vi "TeamLookUP.vi"() -> ()   [LabVIEW 2016]
panel:
  in  "Previous":bool
  in  "Next":bool
  out "Image":T1(plugin-control)
  out "Data":string
  out "Location":string
  out "Name":string
  in  "Done":bool
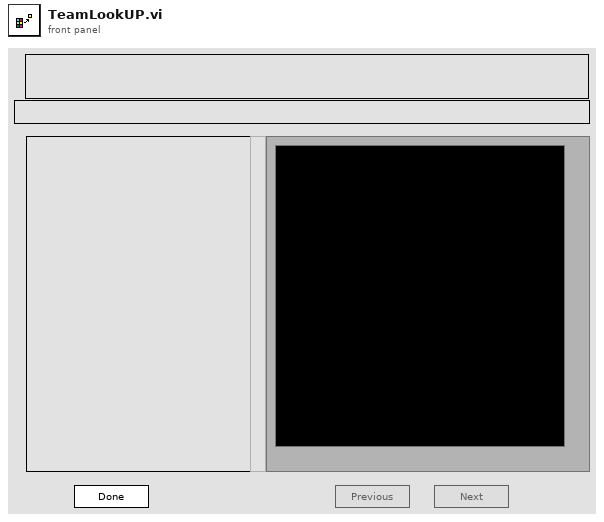
[diagram p1: front panel]
types:
  T1 = typedef "IMAQ Image.ctl" = refnum<image>
  T2 = typedef "Image Type" = u32
  T3 = enum8{"Enabled", "Disabled", "Disabled and Grayed Out"}
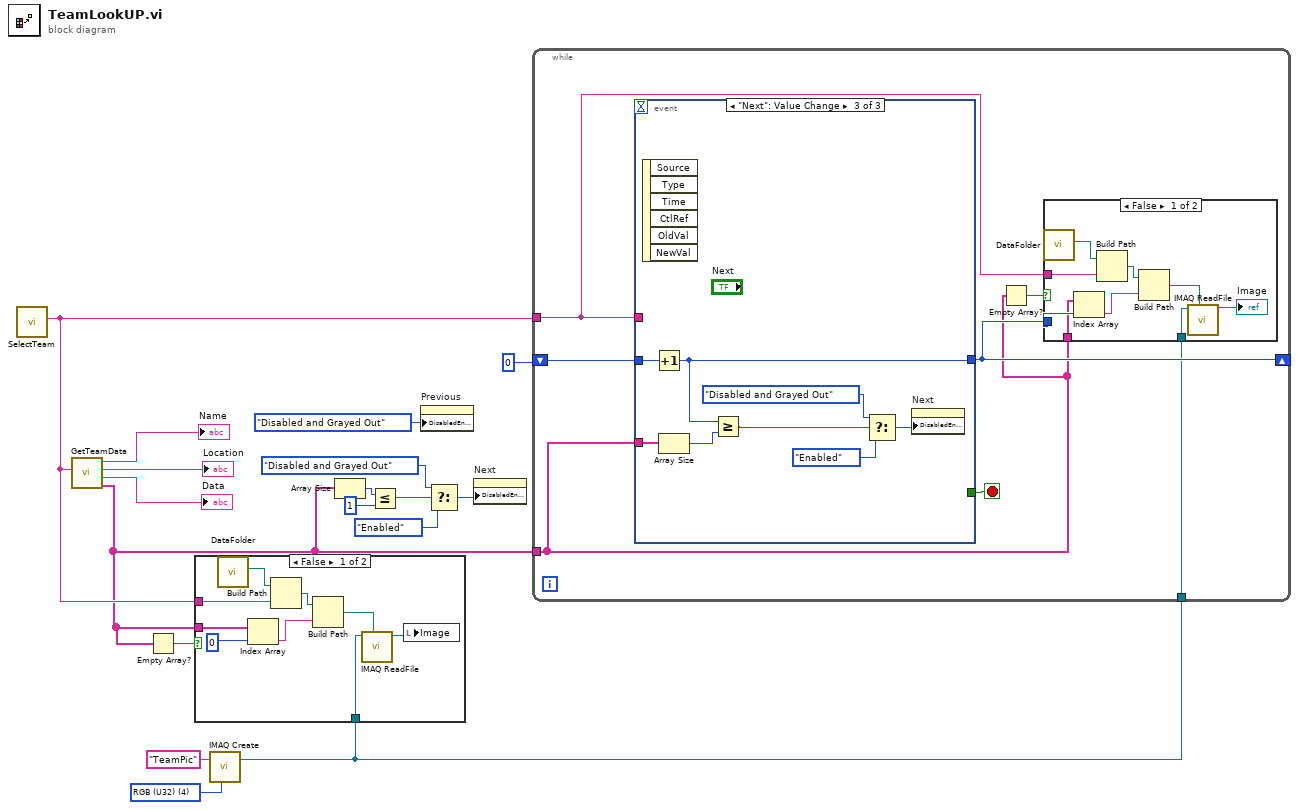
[diagram p0: block diagram]
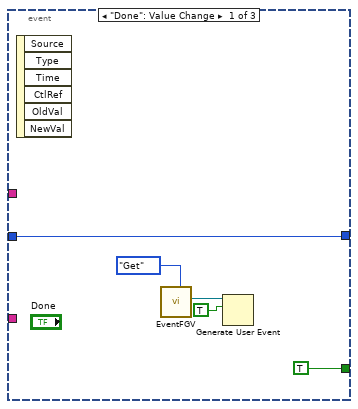
[diagram p4: hidden frame]
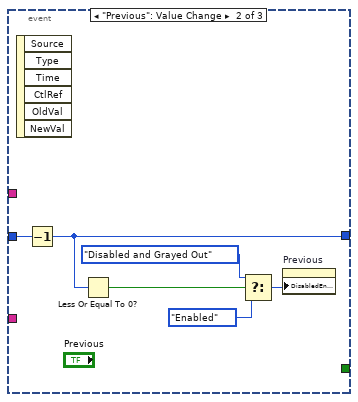
[diagram p5: hidden frame]
diagram:
  w5 = T2 4 items=["Grayscale (U8)", "Grayscale (I16)", "Grayscale (SGL)", "Complex (CSG)", "RGB (U32)", "HSL (U32)", "RGB (U64)", "Grayscale (U16)"] ("Image Type")
  n1 = call "SelectTeam.vi"() -> ("Selected Team"=w4:string)  [unwired: 11 in]
  n2 = call "GetTeamData.vi"("Team #"=w4) -> ("Pictures"=w2:string[], "Data"=→"Data":string, "Location"=→"Location":string, "Name"=→"Name":string)  [unwired: 7 in]
  n3 = Empty Array?(array=w2) -> (empty?=w3:bool)
  n4 = call "IMAQ Create"("Image Name"="TeamPic", "Image Type"=w5) -> ("New Image"=w1:T1)  [unwired: 3 in, 1 out]
  n5 = case shown="False" w3 {
    tunnel: w2 -> [w22 _]
    tunnel: w4 -> [w20 _]
    tunnel: w1 -> [w18 _]
    frame False {
      n6 = call "DataFolder.vi"() -> ("appended path"=w23:path)  [unwired: 11 in]
      n7 = Index Array(array=w22, index=0) -> (element=w25:string)
      n8 = Build Path(base path=w23, name or relative path=w20) -> (appended path=w24:path)
      n9 = Build Path(base path=w24, name or relative path=w25) -> (appended path=w26:path)
      n10 = call "IMAQ ReadFile"("File Path"=w26, "Image"=w18) -> ("Image Out"=w19:T1)  [unwired: 5 in, 4 out]
      n11 = local write "Image"(w19) -> ()
    }
    frame True {
    }
  }
  n12 = Array Size(array=w2) -> (size(s)=w12:i32)
  n13 = Less Or Equal?(x=w12, y=1) -> (x <= y?=w9:bool)
  n14 = property on="Previous" class="Bool"("DisabledEnum"=T3."Disabled and Grayed Out" ("Disabled")) -> ()  [unwired: 2 in, 2 out]
  n15 = Select(t=T3."Disabled and Grayed Out" ("Disabled"), s=w9, f=T3."Enabled" ("Disabled")) -> (s? t:f=w10:T3)
  n16 = property on="Next" class="Bool"("DisabledEnum"=w10) -> ()  [unwired: 2 in, 2 out]
  n17 = while {
    tunnel: w4 -> [w30]
    shift-right: [w31] -> _
    shift-left: 0 -> [w32]
    tunnel: w2 -> [w28]
    tunnel: w1 -> [w29]
    stop <- w33 stop-if-true
    n18 = event shown="[2] \"Next\": Value Change" {
      selector: _ -> [_ _ _]
      dyn-events: _ -> [_ _ _]
      timeout: _ -> [_ _ _]
      tunnel: [TRUE _ _] -> w33
      tunnel: w30 -> [_ _ _]
      tunnel: [w43 w52 w57] -> w31
      tunnel: w32 -> [w43 w53 w61]
      tunnel: w28 -> [_ _ w56]
      event "Done": Value Change {
        n19 = event-data() -> ()  [unwired: 1 in, 6 out]
        n20 = call "EventFGV.vi"("Action"=enum16{"Set", "Get"}."Get") -> ("user event out"=w47:refnum<user-event>)  [unwired: 10 in]
        n21 = Generate User Event(user event=w47, event data cluster=TRUE ("event data")) -> ()  [unwired: 2 in, 2 out]
      }
      event "Previous": Value Change {
        n22 = event-data() -> ()  [unwired: 1 in, 6 out]
        n23 = Decrement(x=w53) -> (x-1=w52:i32)
        n24 = Less Or Equal To 0?(x=w52) -> (x <= 0?=w48:bool)
        n25 = Select(t=T3."Disabled and Grayed Out" ("Disabled"), s=w48, f=T3."Enabled" ("Disabled")) -> (s? t:f=w49:T3)
        n26 = property on="Previous" class="Bool"("DisabledEnum"=w49) -> ()  [unwired: 2 in, 2 out]
      }
      event "Next": Value Change {
        n27 = event-data() -> ()  [unwired: 1 in, 6 out]
        n28 = Increment(x=w61) -> (x+1=w57:i32)
        n29 = Array Size(array=w56) -> (size(s)=w55:i32)
        n30 = Greater Or Equal?(x=w57, y=w55) -> (x >= y?=w54:bool)
        n31 = Select(t=T3."Disabled and Grayed Out" ("Disabled"), s=w54, f=T3."Enabled" ("Disabled")) -> (s? t:f=w58:T3)
        n32 = property on="Next" class="Bool"("DisabledEnum"=w58) -> ()  [unwired: 2 in, 2 out]
      }
    }
    n33 = Empty Array?(array=w28) -> (empty?=w27:bool)
    n34 = case shown="False" w27 {
      tunnel: w31 -> [w42 _]
      tunnel: w28 -> [w41 _]
      tunnel: w30 -> [w39 _]
      tunnel: w29 -> [w34 _]
      frame False {
        n35 = call "DataFolder.vi"() -> ("appended path"=w40:path)  [unwired: 11 in]
        n36 = Index Array(array=w41, index=w42) -> (element=w37:string)
        n37 = Build Path(base path=w40, name or relative path=w39) -> (appended path=w38:path)
        n38 = Build Path(base path=w38, name or relative path=w37) -> (appended path=w35:path)
        n39 = call "IMAQ ReadFile"("File Path"=w35, "Image"=w34) -> ("Image Out"=→"Image":T1)  [unwired: 5 in, 4 out]
      }
      frame True {
      }
    }
  }
